vi "Flyback.vi"() -> ()   [LabVIEW 2014]
uses:
  <vilib>/Analysis/NI_AALBase.lvlib
panel:
  in  "samples":i32=10
  out "XY Graph":cluster{i32[], "sine wave":dbl[]}(graph)
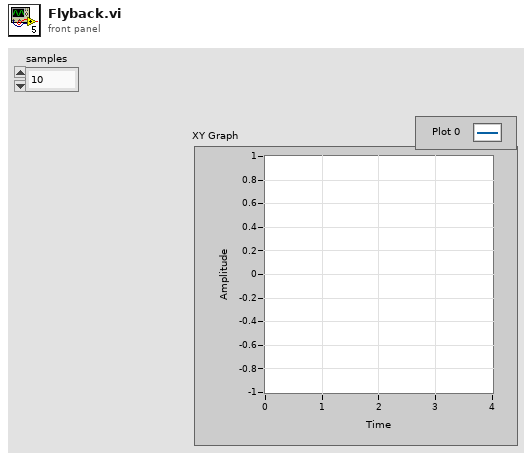
[diagram p1: front panel]
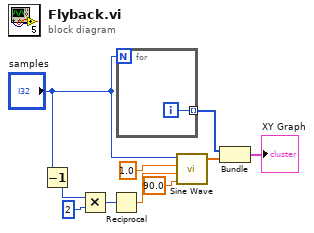
[diagram p0: block diagram]
diagram:
  n1 = Decrement(x="samples") -> (x-1=w1:i32)
  n2 = Multiply(x=w1, y=2) -> (x*y=w4:i32)
  n3 = Reciprocal(x=w4) -> (1/x=w5:dbl)
  n4 = for {
    N: "samples" -> [_]
    tunnel: [w11] -> w9 mode=indexing
    i -> [w11]
  }
  n5 = call <vilib>:"Sine Wave.vi"("samples"="samples", "amplitude"=1.0, "frequency"=w5, "phase in"=90.0) -> ("sine wave"=w8:dbl[])  [unwired: 1 in, 2 out]
  n6 = Bundle(w9, "sine wave"=w8) -> (→"XY Graph":cluster{i32[], "sine wave":dbl[]})  [unwired: 1 in]
